vi "Set Initialization Data - gRPC Server.vi"(8 "error in":errorcluster, 11 "gRPC Server Tester in":refnum<class "gRPC Server Tester.lvclass">) -> (0 "error out":errorcluster, 3 "gRPC Server Tester out":refnum<class "gRPC Server Tester.lvclass">)   [LabVIEW 2019, in "gRPC Server Tester.lvclass"]
doc: "In this VI you can set the initialization data of a statically-linked subWorker."
uses:
  gRPC Server Tester.lvclass
  gRPC Server/gRPC Server/Initialization Data.ctl
  gRPC Server/gRPC Server/Response Cases.ctl
  <vilib>/addons/_Workers/Library/Case Label.ctl
  gRPC Server Tester.lvclass/gRPC Server Tester.ctl
  gRPC Server/gRPC Server/gRPC Server.lvclass
  C:/Program Files (x86)/National Instruments/LabVIEW 2019/vi.lib/addons/_Workers/Library/Classes/Worker/Worker.lvclass
  <vilib>/addons/_Workers/Library/Workers.lvlib
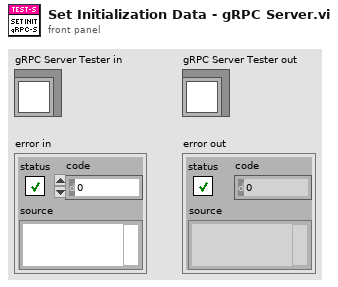
[diagram p1: front panel]
types:
  T1 = typedef "gRPC Server (template.proto).lvlib/gRPC Server.lvclass/Initialization Data.ctl" = cluster{"Response Cases":T2}
  T2 = typedef "gRPC Server (template.proto).lvlib/gRPC Server.lvclass/Response Cases.ctl" = cluster{"Connection Notify":T3, "Server Error":T3, "Msg_ToServer_1":T3, "Msg_ToServer_2":T3, "Msg_ToServer_3":T3, "Msg_ToServer_4":T3, "Msg_ToServer_5":T3, "Msg_ToServer_6":T3, "Msg_ToServer_7":T3, "Msg_ToServer_8":T3, "Msg_ToServer_9":T3}
  T3 = typedef "Workers.lvlib/Case Label.ctl" = string
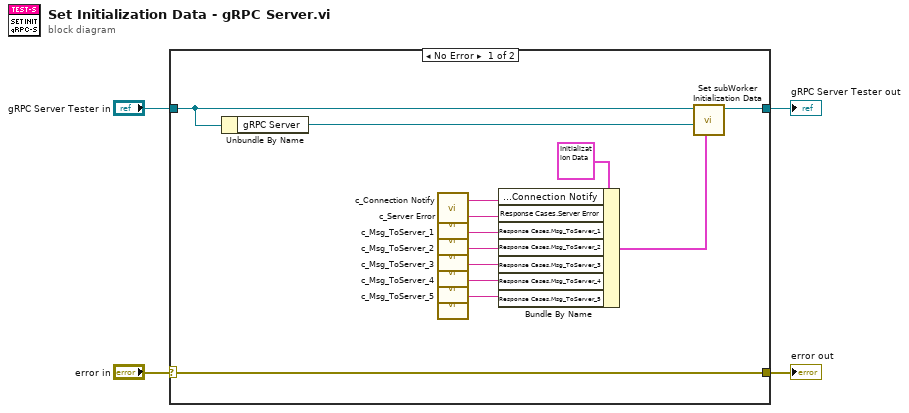
[diagram p0: block diagram]
diagram:
  n1 = case shown="No Error" "error in" {
    selector: "error in" -> [w17 w19]
    tunnel: [w17 w19] -> w3
    tunnel: [w15 w18] -> w2
    tunnel: "gRPC Server Tester in" -> [w14 w18]
    frame No Error {
      n2 = Unbundle By Name(w14) -> ("gRPC Server"=w16:refnum<class "gRPC Server.lvclass">)
      n3 = call "c_Connection Notify.vi"() -> ("Case Label"=w11:T3)  [unwired: 1 in]
      n4 = call "c_Server Error.vi"() -> ("Case Label"=w10:T3)  [unwired: 1 in]
      n5 = call "c_Msg_ToServer_1.vi"() -> ("Case Label"=w9:T3)  [unwired: 1 in]
      n6 = call "c_Msg_ToServer_2.vi"() -> ("Case Label"=w8:T3)  [unwired: 1 in]
      n7 = call "c_Msg_ToServer_3.vi"() -> ("Case Label"=w7:T3)  [unwired: 1 in]
      n8 = call "c_Msg_ToServer_4.vi"() -> ("Case Label"=w6:T3)  [unwired: 1 in]
      n9 = call "c_Msg_ToServer_5.vi"() -> ("Case Label"=w5:T3)  [unwired: 1 in]
      n10 = Bundle By Name(cluster=T1 {"Response Cases"={"Connection Notify"="", "Server Error"="", "Msg_ToServer_1"="", "Msg_ToServer_2"="", "Msg_ToServer_3"="", "Msg_ToServer_4"="", "Msg_ToServer_5"="", "Msg_ToServer_6"="", "Msg_ToServer_7"="", "Msg_ToServer_8"="", "Msg_ToServer_9"=""}} ("Initialization Data"), "Response Cases.Connection Notify"=w11, "Response Cases.Server Error"=w10, "Response Cases.Msg_ToServer_1"=w9, "Response Cases.Msg_ToServer_2"=w8, "Response Cases.Msg_ToServer_3"=w7, "Response Cases.Msg_ToServer_4"=w6, "Response Cases.Msg_ToServer_5"=w5) -> (w12:T1)
      n11 = call-dynamic "Set subWorker Initialization Data.vi"("Initialization Data"=w12, "subWorker"=w16, "Worker"=w14) -> ("Worker out"=w15:refnum<class "gRPC Server Tester.lvclass">)  [unwired: 8 in]
    }
    frame Error {
    }
  }
  "error out" <- w3
  "gRPC Server Tester out" <- w2
